vi "COM Port Initialization.vi"(8 "error in (no error)":errorcluster, 11 "Communication Settings":T1={"Unit ID"="A", "Baud Rate"=enum."19200", "VISA Sesssion In"="COM1"}) -> (0 "error out":errorcluster, 3 "VISA Session Out":refnum<visa-resource-name>)   [LabVIEW 2018]
doc: "Initializes the serial connection to a specified COM port. Baud rate should match the baud rate of the connected Alicat(s). If multiple Alicats are connected to the specified COM port, ensure that they all have unique unit ID's.\n\nThe Unit ID is not used for the initialization step. If connecting to multiple Alicats, leave it as the default \"A\"."
uses:
  <vilib>/Instr/_visa.llb/VISA Open Access Mode.ctl
panel:
  # "Unit ID is not used. If you\nneed to run this with many\nunits, just pass a default ID of \"A\""
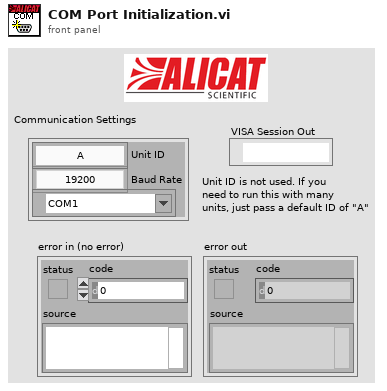
[diagram p1: front panel]
types:
  T1 = cluster{"Unit ID":string, "Baud Rate":enum8{"2400", "9600", "19200", "38400", "57600", "115200", "Unknown"}, "VISA Sesssion In":refnum<visa-resource-name>}
  T2 = enum8{"2400", "9600", "19200", "38400", "57600", "115200", "Unknown"}
  T3 = typedef "VISA Open Access Mode.ctl" = u32
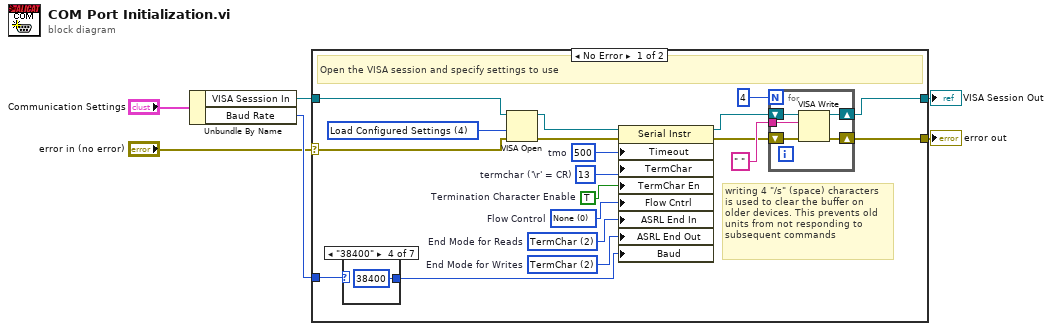
[diagram p0: block diagram]
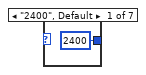
[diagram p2: hidden frame]
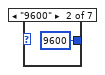
[diagram p3: hidden frame]
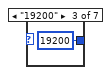
[diagram p4: hidden frame]
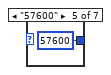
[diagram p5: hidden frame]
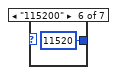
[diagram p6: hidden frame]
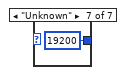
[diagram p7: hidden frame]
diagram:
  n1 = Unbundle By Name("Communication Settings") -> ("VISA Sesssion In"=w1:refnum<visa-resource-name>, "Baud Rate"=w5:T2)
  n2 = case shown="No Error" "error in (no error)" {
    selector: "error in (no error)" -> [w13 w39]
    tunnel: w5 -> [w25 _]
    tunnel: [w8 w38] -> w3
    tunnel: [w7 w39] -> w2
    tunnel: w1 -> [w20 w38]
    frame No Error {
      w21 = T3 4 items=["VISA Defaults"=0, "Exclusive Lock"=1, "Load Configured Settings"=4] ("Access Mode")
      w19 = u32 500  # tmo
      w18 = u16 2 items=["None", "Last Bit", "TermChar", "Break"]  # End Mode for Writes
      w17 = u16 2 items=["None", "Last Bit", "TermChar"]  # End Mode for Reads
      w16 = u16 0 items=["None", "XON/XOFF", "RTS/CTS", "XON/XOFF & RTS/CTS", "DTR/DSR", "XON/XOFF & DTR/DSR"]  # Flow Control
      w15 = TRUE  # Termination Character Enable
      w14 = u8 13  # termchar ('\r' = CR)
      # "writing 4 \"/s\" (space) characters\nis used to clear the buffer on \nolder devices. This prevents old\nunits from not responding to \nsubsequent commands"
      # "Open the VISA session and specify settings to use"
      n3 = case shown="\"38400\"" w25 {
        tunnel: [u32 2400 ("Serial Settings:Baud Rate") u32 9600 ("Serial Settings:Baud Rate") u32 19200 ("Serial Settings:Baud Rate") u32 38400 ("Serial Settings:Baud Rate") u32 57600 ("Serial Settings:Baud Rate") u32 11520 ("Serial Settings:Baud Rate") u32 19200 ("Serial Settings:Baud Rate")] -> w22
        frame "2400", Default {
        }
        frame "9600" {
        }
        frame "19200" {
        }
        frame "38400" {
        }
        frame "57600" {
        }
        frame "115200" {
        }
        frame "Unknown" {
        }
      }
      n4 = VISA Open(access mode=w21, error in (no error)=w13, VISA resource name=w20) -> (VISA resource name=w23:refnum<visa-resource-name>, error out=w24:errorcluster)  [unwired: 2 in]
      n5 = property class="Serial Instr"(reference=w23, error in=w24, "Timeout"=w19, "TermChar"=w14, "TermChar En"=w15, "Flow Cntrl"=w16, "ASRL End In"=w17, "ASRL End Out"=w18, "Baud"=w22) -> (reference out=w9:refnum<visa-resource-name>, error out=w10:errorcluster)
      n6 = for {
        N: 4 -> [_]
        tunnel: " " -> [w26]
        shift-right: [w27] -> w8
        shift-left: w9 -> [w28]
        shift-right: [w29] -> w7
        shift-left: w10 -> [w30]
        n7 = VISA Write(VISA resource name=w28, write buffer=w26, error in (no error)=w30) -> (VISA resource name out=w27:refnum<visa-resource-name>, error out=w29:errorcluster)  [unwired: 1 out]
      }
    }
    frame Error {
    }
  }
  "VISA Session Out" <- w3
  "error out" <- w2
